vi "Engine-Event-MouseButtonDown.vi"(4 "y":sgl, 5 "Clicks":u8, 6 "x":sgl, 7 "Button":u8, 8 "error in (no error)":errorcluster, 9 "Which":T1, 10 "Timestamp":u64, 11 "GLF Window in":refnum<class "Window.lvclass">) -> (0 "error out":errorcluster, 3 "GLF Window out":refnum<class "Window.lvclass">)   [LabVIEW 2020, in "GLF.lvlib" / "Window.lvclass"]
uses:
  Window.lvclass
  Window.lvclass/Window.ctl
  WindowEventInterface/WindowEventInterface.lvclass
  <vilib>/Saukko/LV SDL3/Sources/SDL3/Mouse/MouseID--integer.ctl
  <vilib>/Saukko/LV SDL3/Sources/SDL3/Mouse/Mouse.lvlib
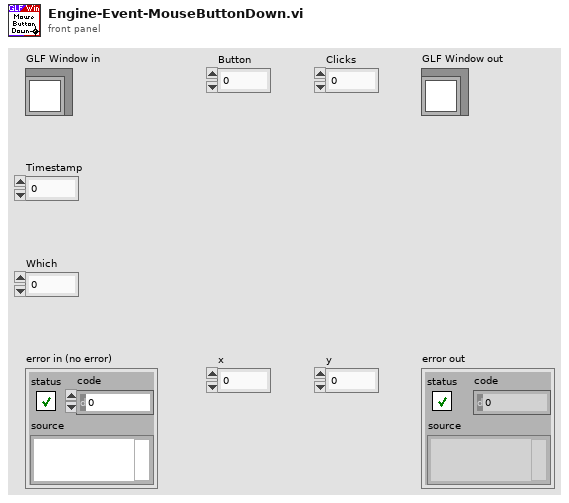
[diagram p1: front panel]
types:
  T1 = typedef "SDL3.lvlib/Mouse.lvlib/MouseID--integer.ctl" = u32
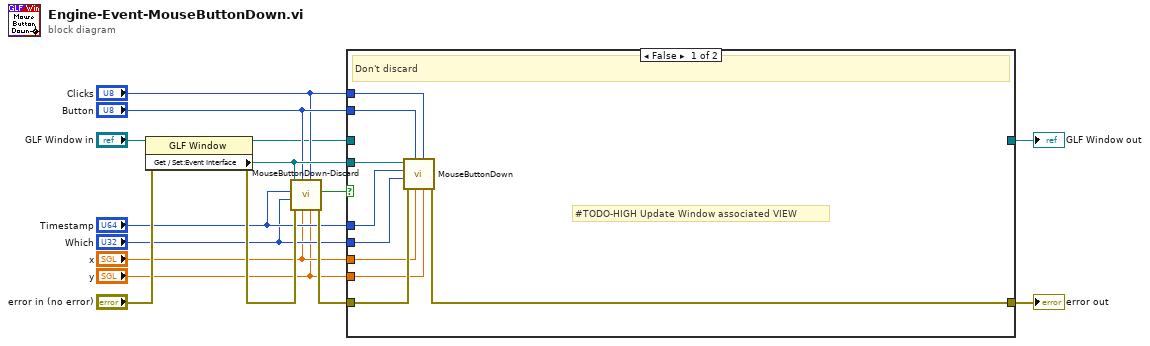
[diagram p0: block diagram]
diagram:
  n1 = property class="GLF Window"(reference="GLF Window in", error in="error in (no error)") -> (reference out=w2:refnum<class "Window.lvclass">, error out=w13:errorcluster, "Get / Set:Event Interface"=w10:refnum<class "WindowEventInterface.lvclass">)
  n2 = call-dynamic "MouseButtonDown-Discard.vi"("y"="y", "Clicks"="Clicks", "x"="x", "Button"="Button", "error in (no error)"=w13, "Which"="Which", "Timestamp"="Timestamp", "WindowEventInterface in"=w10) -> ("error out"=w12:errorcluster, "Discard?"=w3:bool)  [unwired: 2 in]
  n3 = case shown="False" w3 {
    tunnel: [w24 w25] -> w14
    tunnel: w12 -> [w23 w25]
    tunnel: w10 -> [w22 _]
    tunnel: "Button" -> [w21 _]
    tunnel: "Clicks" -> [w20 _]
    tunnel: "Timestamp" -> [w19 _]
    tunnel: "Which" -> [w18 _]
    tunnel: "x" -> [w17 _]
    tunnel: "y" -> [w16 _]
    tunnel: w2 -> [_ w26]
    tunnel: [_ w26] -> w1
    frame False {
      # "#TODO-HIGH Update Window associated VIEW"
      # "Don't discard"
      n4 = call-dynamic "MouseButtonDown.vi"("y"=w16, "Clicks"=w20, "x"=w17, "Button"=w21, "error in (no error)"=w23, "Which"=w18, "Timestamp"=w19, "WindowEventInterface in"=w22) -> ("error out"=w24:errorcluster)  [unwired: 3 in]
    }
    frame True {
      # "Discard"
    }
  }
  "error out" <- w14
  "GLF Window out" <- w1
